vi "ReplaceArraySubset.vi"() -> ()   [LabVIEW 2019]
panel:
  out "output array 2":dbl[](array[numeric])
  out "output array":dbl[](array[numeric])
  in  "Array":dbl[](array[numeric])=[10.0, 20.0, 30.0, 40.0]
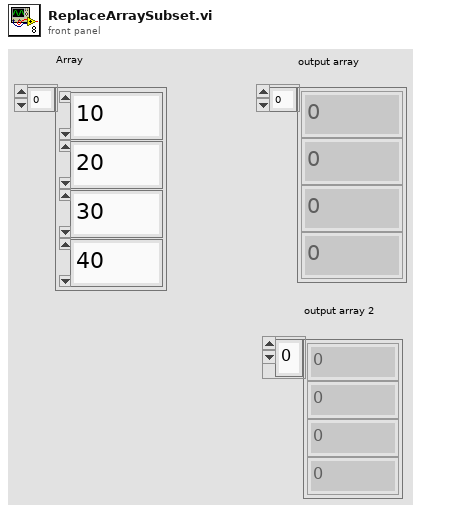
[diagram p1: front panel]
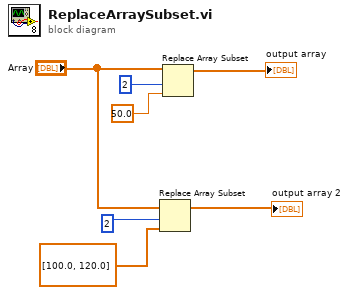
[diagram p0: block diagram]
diagram:
  n1 = Replace Array Subset(array="Array", new element=dbl[] [100.0, 120.0], index=2) -> (→"output array 2":dbl[])
  n2 = Replace Array Subset(array="Array", new element=50.0 ("new element/subarray"), index=2) -> (→"output array":dbl[])
